vi "Test AI.vi"() -> ()   [LabVIEW 2009, in "MicroDAQ.lvlib"]
uses:
  <instrlib>/MicroDAQ/MicroDAQ.lvlib
  <instrlib>/MicroDAQ/Temp Tests/Test AI enum.ctl
  <instrlib>/MicroDAQ/Tools/Analog input type enum.ctl
  <instrlib>/MicroDAQ/Tools/Analog input Channel enum.ctl
  <instrlib>/MicroDAQ/Tools/Analo Range Enum.ctl
  <instrlib>/MicroDAQ/Channel/Analog Input/Read NChan NSamp 2D SGL.vi
  <instrlib>/MicroDAQ/Channel/Analog Input/AI Configure Channel.vi
  <instrlib>/MicroDAQ/Channel/Analog Input/Analog Input.lvclass
  <instrlib>/MicroDAQ/Channel/Analog Input/Read 1Chan 1Samp 1D SGL.vi
  <instrlib>/MicroDAQ/Tools/Analog Channel Enum.ctl
  <instrlib>/MicroDAQ/Channel/Analog Output/Write 1Chan 1Sample SGL.vi
  <instrlib>/MicroDAQ/Channel/Analog Output/Analog output.lvclass
  <instrlib>/MicroDAQ/Tools/Analog mode.ctl
  <instrlib>/MicroDAQ/Channel/Analog Output/Write NChan 1Sample 1D SGL.vi
  <instrlib>/MicroDAQ/Channel/Analog Output/Write NChan NSamp 2D SGL.vi
  <instrlib>/MicroDAQ/Channel/Analog Output/AO Configure Channel.vi
  <instrlib>/MicroDAQ/MLink32.dll
panel:
  out "Value":dbl
  out "Waveform Chart":dbl[][](graph)
  out "read samples":i32
  out "Current Test":T1
  in  "Test to execute":T1[](array[typedef])=[enum."Default Config Read NChan NSamp", enum."Default Config Read 1Chan 1Sample", enum."Default Config Read 1Chan 1Sample (with Start)"]
  out "error occured":errorcluster
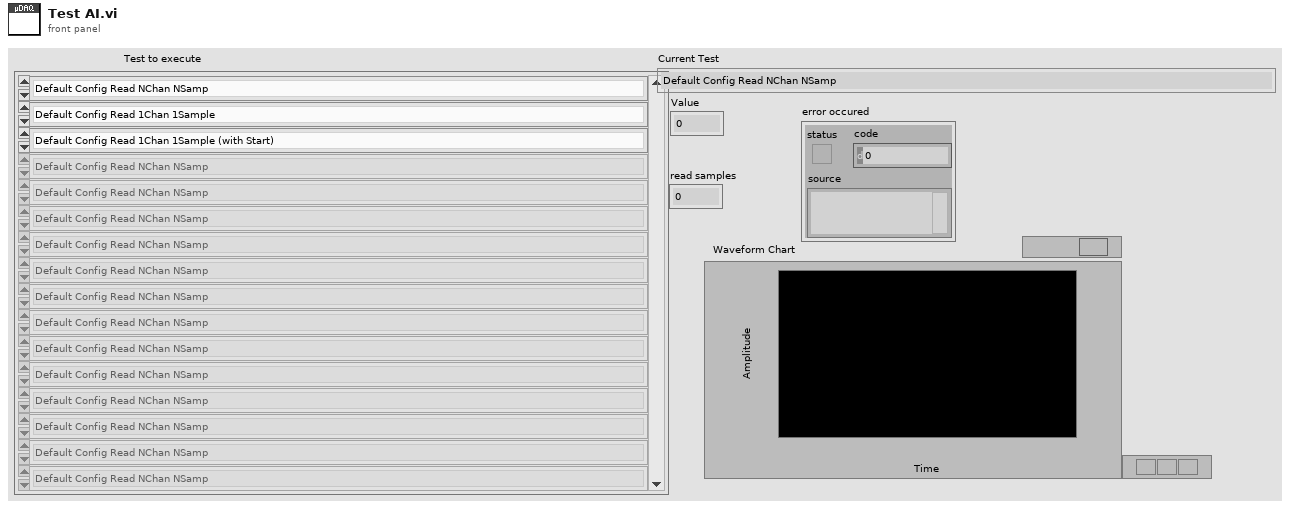
[diagram p1: front panel]
types:
  T1 = typedef "MicroDAQ.lvlib/Test AI enum.ctl" = enum16{"Default Config Read NChan NSamp", "Default Config Read 1Chan 1Sample", "Default Config Read 1Chan 1Sample (with Start)", "Default Config 2Chan NSamp followed by Read 1Samp", "Default Config 2Chan NSamp followed by Read 1Samp followed by Read NSamp"}
  T2 = typedef "MicroDAQ.lvlib/Analog mode.ctl" = enum16{"Periodic", "Stream"}
  T3 = typedef "MicroDAQ.lvlib/Analog input type enum.ctl" = enum16{"Single-ended", "Differential"}
  T4 = typedef "MicroDAQ.lvlib/Analog input Channel enum.ctl" = enum16{"None", "AI1", "AI2", "AI3", "AI4", "AI5", "AI6", "AI7", "AI8", "AI9", "AI10", "AI11", "AI12", "AI13", "AI14", "AI15", "AI16"}
  T5 = typedef "MicroDAQ.lvlib/Analo Range Enum.ctl" = enum16{"±10V", "0-10V", "±5V", "0-5V", "±5.12V", "±2.56V", "±2.5V", "±2V", "±1.24V", "±0.64V"}
  T6 = typedef "MicroDAQ.lvlib/Analog Channel Enum.ctl" = enum16{"None", "AO1", "AO2", "AO3", "AO4", "AO5", "AO6", "AO7", "AO8", "AO9", "AO10", "AO11", "AO12", "AO13", "AO14", "AO15", "AO16"}
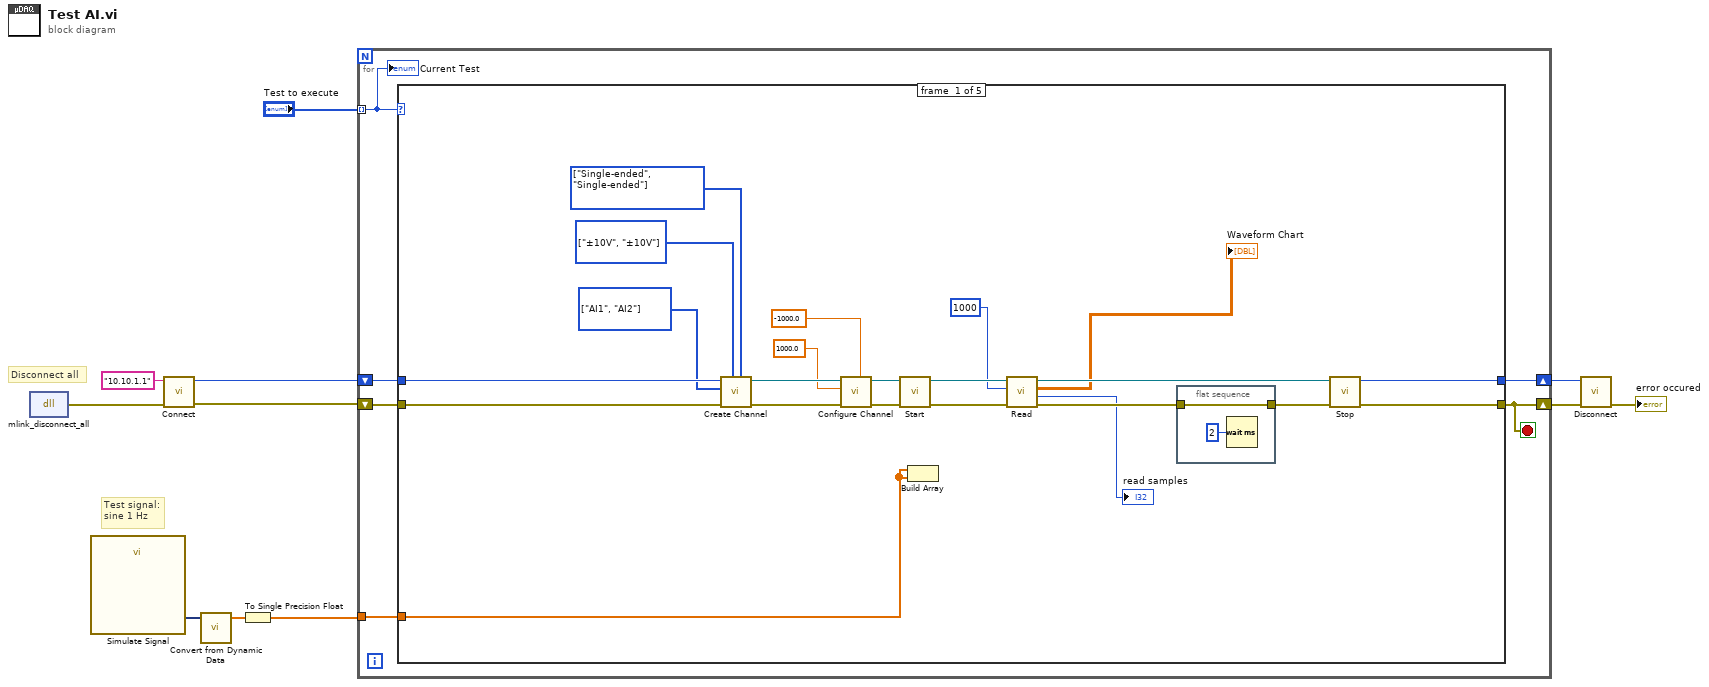
[diagram p0: block diagram]
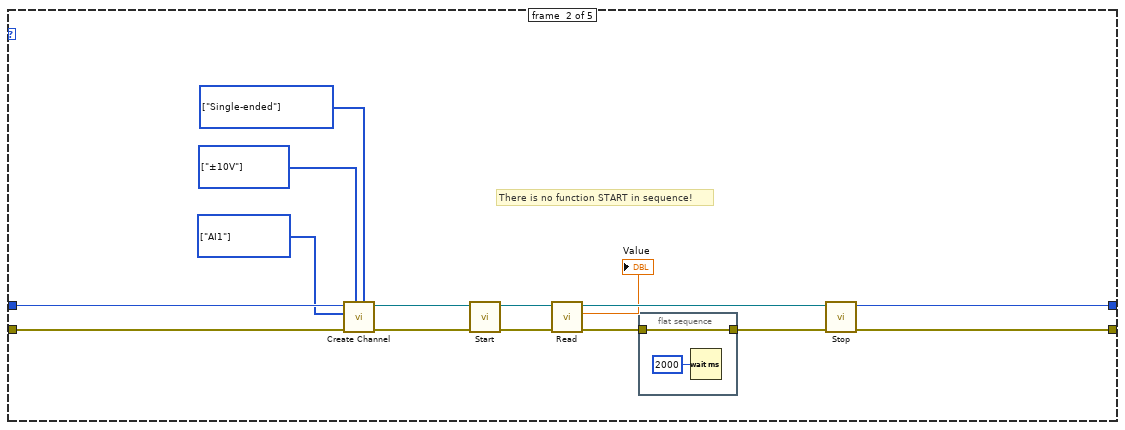
[diagram p2: hidden frame]
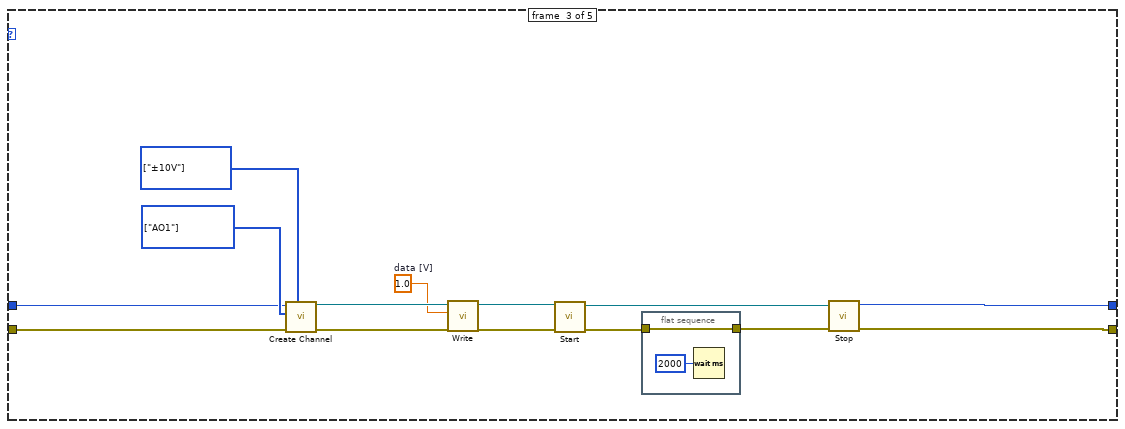
[diagram p3: hidden frame]
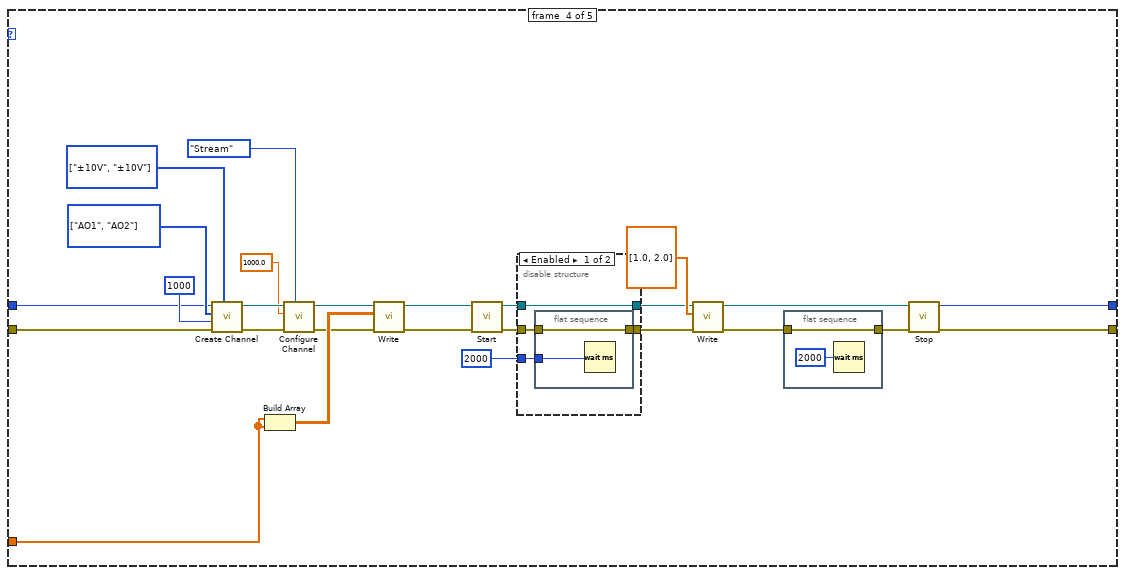
[diagram p4: hidden frame]
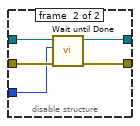
[diagram p5: hidden frame]
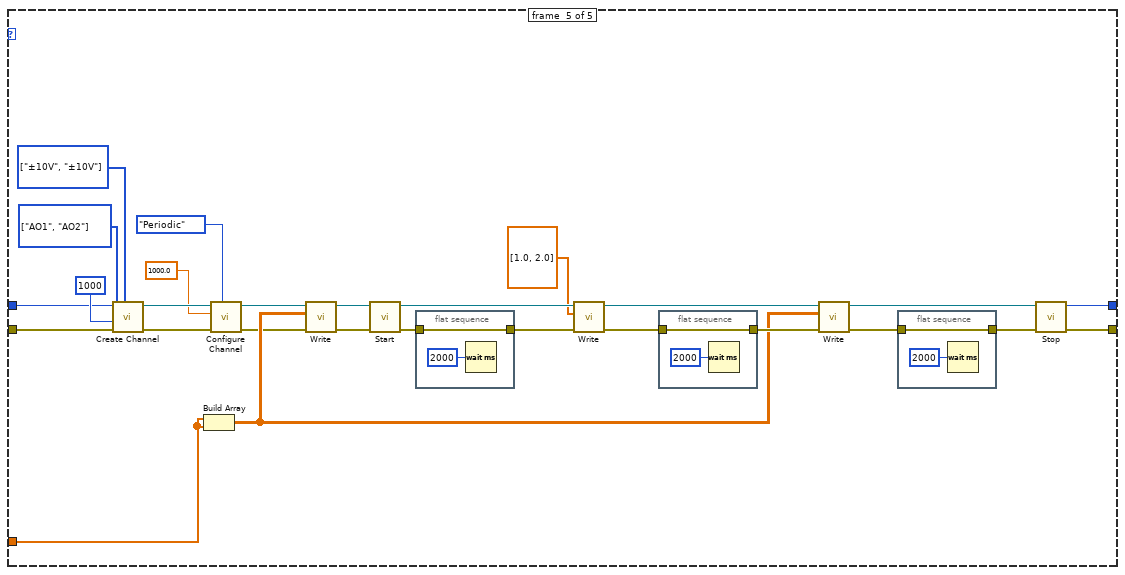
[diagram p6: hidden frame]
diagram:
  # "Test signal:\nsine 1 Hz"
  # "Disconnect all"
  n1 = dll-call lib="C:/Program Files (x86)/National Instruments/LabVIEW 2009/instr.lib/MicroDAQ/MLink32.dll" fn="mlink_disconnect_all" ("MLink32.*:mlink_connect")() -> (error out=w11:errorcluster)  [unwired: 4 in, 1 out]
  n2 = call "Simulate Signal"() -> ("Sine"=w7:dynamicdata)  [unwired: 14 in, 1 out]
  n3 = call <instrlib>:"Connect.vi"("error in (no error)"=w11, "IP address"="10.10.1.1") -> ("error out"=w9:errorcluster, "connection ID"=w10:i32)  [unwired: 8 in]
  n4 = call "Convert from Dynamic Data"("Dynamic Data Type"=w7) -> ("Array"=w6:dbl[])  [unwired: 3 in]
  n5 = To Single Precision Float(number=w6) -> (single precision float=w5:sgl[])
  n6 = for {
    tunnel: w5 -> [w15]
    tunnel: "Test to execute" -> [w14] mode=indexing
    shift-right: [w13] -> w3
    shift-left: w10 -> [w17]
    shift-right: [w12] -> w2
    shift-left: w9 -> [w16]
    stop <- w12 stop-if-true
    n7 = case shown="\"Default Config Read 1Chan 1Sample\"" w14 {
      tunnel: w17 -> [w39 w55 w66 w85 w130]
      tunnel: w16 -> [w38 w54 w65 w84 w129]
      tunnel: w15 -> [w36 _ _ w88 w128]
      tunnel: [w33 w50 w63 w90 w123] -> w12
      tunnel: [w32 w49 w64 w89 w124] -> w13
      frame #0 {
        w20 = T3[] [enum."Single-ended", enum."Single-ended"] items=["Single-ended", "Differential"] ("Input terminals configurations")
        w27 = T4[] [enum."AI1", enum."AI2"] items=["None", "AI1", "AI2", "AI3", "AI4", "AI5", "AI6", "AI7", "AI8", "AI9", "AI10", "AI11", "AI12", "AI13", "AI14", "AI15", "AI16"] ("Phisical channels")
        w37 = T5[] [enum."±10V", enum."±10V"] items=["±10V", "0-10V", "±5V", "0-5V", "±5.12V", "±2.56V", "±2.5V", "±2V", "±1.24V", "±0.64V"] ("ranges")
        # "AO Basic Config Write (2s) test, 2 Channels"
        n8 = call-poly <instrlib>:"Create Channel.vi"("Input terminals configurations"=w20, "Ranges"=w37, "error in (no error)"=w38, "Phisical channels"=w27, "connection ID"=w39) -> ("error out"=w31:errorcluster, "Task Out"=w30:refnum<class "Analog Input.lvclass">)  [unwired: 5 in]
        n9 = call-poly <instrlib>:"Configure Channel.vi"("Samples per channel"=-1000.0, "error in (no error)"=w31, "Sampe Rate"=1000.0, "MicroDAQ.lvlib:Analog Input.lvclass"=w30) -> ("error out"=w26:errorcluster, "MicroDAQ.lvlib:Analog Input.lvclass out"=w25:refnum<class "Analog Input.lvclass">)  [unwired: 6 in]
        n10 = call-dynamic "Start.vi"("error in (no error)"=w26, "Analog Input in"=w25) -> ("error out"=w23:errorcluster, "Analog Input out"=w34:refnum<class "Analog Input.lvclass">)  [unwired: 8 in]
        n11 = Build Array(w36, w36) -> ()  [unwired: 1 out]
        n12 = call-poly <instrlib>:"Read.vi"("error in (no error)"=w23, "number of samples per channel"=1000, "MicroDAQ.lvlib:Analog Input.lvclass"=w34) -> ("error out"=w22:errorcluster, "read samples"=→"read samples":i32, "Values"=→"Waveform Chart":dbl[][], "MicroDAQ.lvlib:Analog Input.lvclass out"=w24:refnum<class "Analog Input.lvclass">)  [unwired: 5 in]
        n13 = flat-sequence {
          tunnel: w22 -> [w40]
          tunnel: [w40] -> w35
          frame #0 {
            n14 = Wait (ms)(milliseconds to wait=u32 2) -> ()  [unwired: 1 out]
          }
        }
        n15 = call-dynamic "Stop.vi"("error in (no error)"=w35, "Analog Input in"=w24) -> ("error out"=w33:errorcluster, "connection ID"=w32:i32)  [unwired: 8 in]
      }
      frame #1 {
        w46 = T3[] [enum."Single-ended"] items=["Single-ended", "Differential"] ("Input terminals configurations")
        w48 = T4[] [enum."AI1"] items=["None", "AI1", "AI2", "AI3", "AI4", "AI5", "AI6", "AI7", "AI8", "AI9", "AI10", "AI11", "AI12", "AI13", "AI14", "AI15", "AI16"] ("Phisical channels")
        w56 = T5[] [enum."±10V"] items=["±10V", "0-10V", "±5V", "0-5V", "±5.12V", "±2.56V", "±2.5V", "±2V", "±1.24V", "±0.64V"] ("ranges")
        # "There is no function START in sequence!"
        n16 = call-poly <instrlib>:"Create Channel.vi"("Input terminals configurations"=w46, "Ranges"=w56, "error in (no error)"=w54, "Phisical channels"=w48, "connection ID"=w55) -> ("error out"=w42:errorcluster, "Task Out"=w45:refnum<class "Analog Input.lvclass">)  [unwired: 5 in]
        n17 = call-dynamic "Start.vi"("error in (no error)"=w42, "Analog Input in"=w45) -> ("error out"=w43:errorcluster, "Analog Input out"=w44:refnum<class "Analog Input.lvclass">)  [unwired: 8 in]
        n18 = call-poly <instrlib>:"Read.vi"("error in (no error)"=w43, "MicroDAQ.lvlib:Analog Input.lvclass"=w44) -> ("error out"=w52:errorcluster, "Value"=→"Value":dbl, "MicroDAQ.lvlib:Analog Input.lvclass out"=w53:refnum<class "Analog Input.lvclass">)  [unwired: 7 in]
        n19 = flat-sequence {
          tunnel: w52 -> [w57]
          tunnel: [w57] -> w51
          frame #0 {
            n20 = Wait (ms)(milliseconds to wait=u32 2000) -> ()  [unwired: 1 out]
          }
        }
        n21 = call-dynamic "Stop.vi"("error in (no error)"=w51, "Analog Input in"=w53) -> ("error out"=w50:errorcluster, "connection ID"=w49:i32)  [unwired: 8 in]
      }
      frame #2 {
        w68 = sgl 1.0  # data [V]
        w71 = T6[] [enum."AO1"] items=["None", "AO1", "AO2", "AO3", "AO4", "AO5", "AO6", "AO7", "AO8", "AO9", "AO10", "AO11", "AO12", "AO13", "AO14", "AO15", "AO16"] ("channels")
        w72 = T5[] [enum."±10V"] items=["±10V", "0-10V", "±5V", "0-5V", "±5.12V", "±2.56V", "±2.5V", "±2V", "±1.24V", "±0.64V"] ("ranges")
        n22 = call-poly <instrlib>:"Create Channel.vi"("Ranges"=w72, "error in (no error)"=w65, "Phisical channels"=w71, "Connection ID"=w66) -> ("error out"=w69:errorcluster, "Task Out"=w70:refnum<class "Analog output.lvclass">)  [unwired: 6 in]
        n23 = call-poly <instrlib>:"Write.vi"("error in (no error)"=w69, "data"=w68, "Analog Output in"=w70) -> ("error out"=w62:errorcluster, "Analog Output out"=w61:refnum<class "Analog output.lvclass">)  [unwired: 7 in]
        n24 = call-dynamic "Start.vi"("error in (no error)"=w62, "Analog Output in"=w61) -> ("error out"=w59:errorcluster, "Analog Output out"=w60:refnum<class "Analog output.lvclass">)  [unwired: 8 in]
        n25 = flat-sequence {
          tunnel: w59 -> [w73]
          tunnel: [w73] -> w67
          frame #0 {
            n26 = Wait (ms)(milliseconds to wait=u32 2000) -> ()  [unwired: 1 out]
          }
        }
        n27 = call-dynamic "Stop.vi"("error in (no error)"=w67, "Analog Output in"=w60) -> ("error out"=w63:errorcluster, "connection ID"=w64:i32)  [unwired: 8 in]
      }
      frame #3 {
        w99 = T6[] [enum."AO1", enum."AO2"] items=["None", "AO1", "AO2", "AO3", "AO4", "AO5", "AO6", "AO7", "AO8", "AO9", "AO10", "AO11", "AO12", "AO13", "AO14", "AO15", "AO16"] ("channels")
        w100 = T5[] [enum."±10V", enum."±10V"] items=["±10V", "0-10V", "±5V", "0-5V", "±5.12V", "±2.56V", "±2.5V", "±2V", "±1.24V", "±0.64V"] ("ranges")
        n28 = call-poly <instrlib>:"Create Channel.vi"("Ranges"=w100, "error in (no error)"=w84, "Buffer size"=1000 ("buffor size"), "Phisical channels"=w99, "Connection ID"=w85) -> ("error out"=w82:errorcluster, "Task Out"=w83:refnum<class "Analog output.lvclass">)  [unwired: 5 in]
        n29 = Build Array(w88, w88) -> (w87:sgl[][])
        n30 = call-poly <instrlib>:"Configure Channel.vi"("Mode"=Analog_mode."Stream", "error in (no error)"=w82, "Sample rate"=1000.0, "Analog Output in"=w83) -> ("error out"=w81:errorcluster, "Analog Output out"=w80:refnum<class "Analog output.lvclass">)  [unwired: 6 in]
        n31 = call-poly <instrlib>:"Write.vi"("error in (no error)"=w81, "data"=w87, "Analog Output in"=w80) -> ("error out"=w96:errorcluster, "Analog Output out"=w97:refnum<class "Analog output.lvclass">)  [unwired: 7 in]
        n32 = call-dynamic "Start.vi"("error in (no error)"=w96, "Analog Output in"=w97) -> ("error out"=w95:errorcluster, "Analog Output out"=w78:refnum<class "Analog output.lvclass">)  [unwired: 8 in]
        n33 = disable-structure shown="Enabled" {
          disable-tunnel: w95 -> [w104 w111]
          disable-tunnel: [w103 w108] -> w94
          disable-tunnel: w78 -> [w102 w110]
          disable-tunnel: [w102 w109] -> w77
          disable-tunnel: u32 2000 ("milliseconds to wait") -> [w101 w107]
          frame #0 {
            n34 = flat-sequence {
              tunnel: w104 -> [w106]
              tunnel: [w106] -> w103
              tunnel: w101 -> [w105]
              frame #0 {
                n35 = Wait (ms)(milliseconds to wait=w105) -> ()  [unwired: 1 out]
              }
            }
          }
          frame #1 {
            n36 = call-dynamic "Wait until Done.vi"("error in (no error)"=w111, "timeout [s]"=w107, "Analog output in"=w110) -> ("error out"=w108:errorcluster, "Analog output out"=w109:refnum<class "Analog output.lvclass">)  [unwired: 7 in]
          }
        }
        n37 = call-poly <instrlib>:"Write.vi"("error in (no error)"=w94, "data"=dbl[] [1.0, 2.0], "Analog Output in"=w77) -> ("error out"=w93:errorcluster, "Analog Output out"=w92:refnum<class "Analog output.lvclass">)  [unwired: 7 in]
        n38 = flat-sequence {
          tunnel: w93 -> [w112]
          tunnel: [w112] -> w91
          frame #0 {
            n39 = Wait (ms)(milliseconds to wait=u32 2000) -> ()  [unwired: 1 out]
          }
        }
        n40 = call-dynamic "Stop.vi"("error in (no error)"=w91, "Analog Output in"=w92) -> ("error out"=w90:errorcluster, "connection ID"=w89:i32)  [unwired: 8 in]
      }
      frame #4 {
        w139 = T6[] [enum."AO1", enum."AO2"] items=["None", "AO1", "AO2", "AO3", "AO4", "AO5", "AO6", "AO7", "AO8", "AO9", "AO10", "AO11", "AO12", "AO13", "AO14", "AO15", "AO16"] ("channels")
        w140 = T5[] [enum."±10V", enum."±10V"] items=["±10V", "0-10V", "±5V", "0-5V", "±5.12V", "±2.56V", "±2.5V", "±2V", "±1.24V", "±0.64V"] ("ranges")
        n41 = call-poly <instrlib>:"Create Channel.vi"("Ranges"=w140, "error in (no error)"=w129, "Buffer size"=1000 ("buffor size"), "Phisical channels"=w139, "Connection ID"=w130) -> ("error out"=w118:errorcluster, "Task Out"=w119:refnum<class "Analog output.lvclass">)  [unwired: 5 in]
        n42 = Build Array(w128, w128) -> (w122:sgl[][])
        n43 = call-poly <instrlib>:"Configure Channel.vi"("Mode"=Analog_mode."Periodic", "error in (no error)"=w118, "Sample rate"=1000.0, "Analog Output in"=w119) -> ("error out"=w117:errorcluster, "Analog Output out"=w116:refnum<class "Analog output.lvclass">)  [unwired: 6 in]
        n44 = call-poly <instrlib>:"Write.vi"("error in (no error)"=w117, "data"=w122, "Analog Output in"=w116) -> ("error out"=w136:errorcluster, "Analog Output out"=w137:refnum<class "Analog output.lvclass">)  [unwired: 7 in]
        n45 = call-dynamic "Start.vi"("error in (no error)"=w136, "Analog Output in"=w137) -> ("error out"=w135:errorcluster, "Analog Output out"=w132:refnum<class "Analog output.lvclass">)  [unwired: 8 in]
        n46 = flat-sequence {
          tunnel: w135 -> [w145]
          tunnel: [w145] -> w134
          frame #0 {
            n47 = Wait (ms)(milliseconds to wait=u32 2000) -> ()  [unwired: 1 out]
          }
        }
        n48 = call-poly <instrlib>:"Write.vi"("error in (no error)"=w134, "data"=sgl[] [1.0, 2.0], "Analog Output in"=w132) -> ("error out"=w133:errorcluster, "Analog Output out"=w127:refnum<class "Analog output.lvclass">)  [unwired: 7 in]
        n49 = flat-sequence {
          tunnel: w133 -> [w143]
          tunnel: [w143] -> w126
          frame #0 {
            n50 = Wait (ms)(milliseconds to wait=u32 2000) -> ()  [unwired: 1 out]
          }
        }
        n51 = call-poly <instrlib>:"Write.vi"("error in (no error)"=w126, "data"=w122, "Analog Output in"=w127) -> ("error out"=w121:errorcluster, "Analog Output out"=w125:refnum<class "Analog output.lvclass">)  [unwired: 7 in]
        n52 = flat-sequence {
          tunnel: w121 -> [w141]
          tunnel: [w141] -> w120
          frame #0 {
            n53 = Wait (ms)(milliseconds to wait=u32 2000) -> ()  [unwired: 1 out]
          }
        }
        n54 = call-dynamic "Stop.vi"("error in (no error)"=w120, "Analog Output in"=w125) -> ("error out"=w123:errorcluster, "connection ID"=w124:i32)  [unwired: 8 in]
      }
    }
    "Current Test" <- w14
  }
  n55 = call <instrlib>:"Disconnect.vi"("error in (no error)"=w2, "connection ID"=w3) -> ("error out"=→"error occured":errorcluster)  [unwired: 9 in]
